vi "Untitled 3.vi"() -> ()   [LabVIEW 2018]
panel:
  out "Numeric":dbl
  in  "Buttons":bool[](array[boolean])
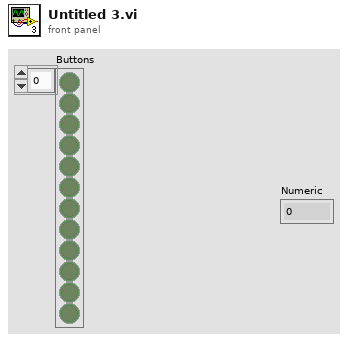
[diagram p1: front panel]
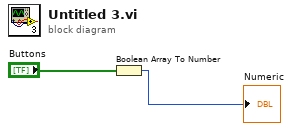
[diagram p0: block diagram]
diagram:
  n1 = Boolean Array To Number(Boolean array="Buttons") -> (number=→"Numeric":u32)
